vi "Procedure - Clear Lines.vi"(11 "error in (no error)":errorcluster, 13 "Socket Mask":u32) -> (15 "error out":errorcluster)   [LabVIEW 2017, in "FPGA-SRL.lvlib"]
uses:
  FPGA-SRL.lvlib
  Type Defs/Write Line Enum.ctl
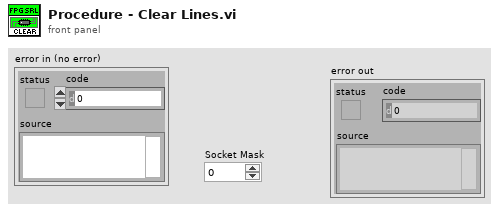
[diagram p1: front panel]
types:
  T1 = typedef "FPGA-SRL.lvlib/Write Line Enum.ctl" = enum16{"DIN", "SYNC", "SCLK"}
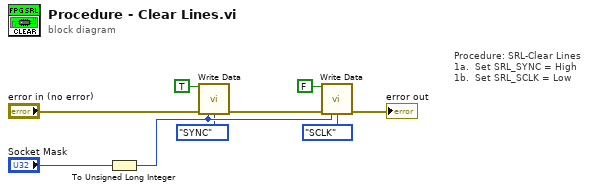
[diagram p0: block diagram]
diagram:
  # "Procedure: SRL-Clear Lines\n1a.  Set SRL_SYNC = High\n1b.  Set SRL_SCLK = Low"
  n1 = To Unsigned Long Integer(number="Socket Mask") -> (unsigned 32bit integer=w7:u32)
  n2 = call "Write Data.vi"("Bit In (SCLK & SYNC)"=TRUE, "error in (no error)"="error in (no error)", "Socket Mask"=w7, "Line"=Write_Line_Enum."SYNC") -> ("error out"=w3:errorcluster)  [unwired: 11 in]
  n3 = call "Write Data.vi"("Bit In (SCLK & SYNC)"=FALSE ("Bit In"), "error in (no error)"=w3, "Socket Mask"=w7, "Line"=Write_Line_Enum."SCLK") -> ("error out"=→"error out":errorcluster)  [unwired: 11 in]
